vi "Index_Read.vi"(8 "error in (no error)":errorcluster) -> (0 "error out":errorcluster, 2 "Found?":bool, 3 "Index":T1)   [LabVIEW 2016, in "SeqProcessor.lvlib"]
uses:
  SeqProcessor.lvlib
  controls/StepIndex.ctl
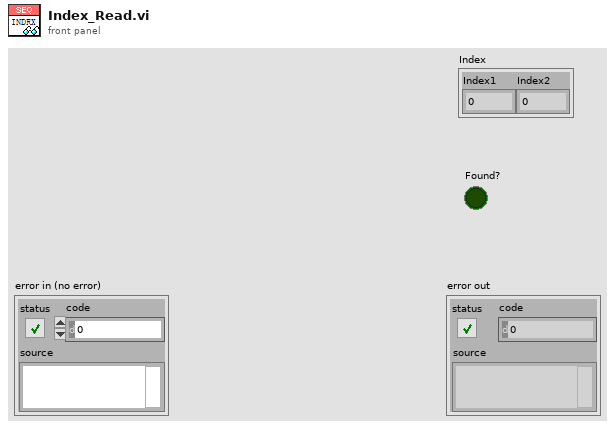
[diagram p1: front panel]
types:
  T1 = typedef "SeqProcessor.lvlib/StepIndex.ctl" = cluster{"Index1":u32, "Index2":u32}
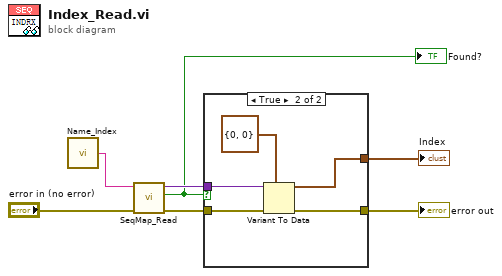
[diagram p0: block diagram]
diagram:
  n1 = call "Name_Index.vi"() -> ("StepIndex"=w3:string)  [unwired: 5 in]
  n2 = call "SeqMap_Read.vi"("error in (no error)"="error in (no error)", "Tag"=w3) -> ("Error Out"=w4:errorcluster, "Found?"=w1:bool, "Value"=w2:variant)  [unwired: 7 in]
  "Found?" <- w1
  n3 = case shown="True" w1 {
    tunnel: w4 -> [w8 w13]
    tunnel: [w8 w12] -> w7
    tunnel: w2 -> [_ w11]
    tunnel: [_ w10] -> w6
    frame False {
    }
    frame True {
      n4 = Variant To Data(error in=w13, type=T1 {"Index1"=0, "Index2"=0} ("Index"), Variant=w11) -> (data=w10:T1, error out=w12:errorcluster)
    }
  }
  "error out" <- w7
  "Index" <- w6
